vi "Calc_orders_FP.vi"() -> ()   [LabVIEW 2010]
panel:
  out "Phi Internal(deg)":dbl
  out "Pix rad (first ring)":dbl
  out "PhiExterna (deg)":dbl
  out "PhiExterna (rad)":dbl
  out "Phi Internal(rad)":dbl
  in  "order in":dbl=1100.0
  out "Angle (deg) cal-ed":dbl=9.9609375
  in  "rad first rimngs\n (pixels)":dbl=600.0
  out "gap (microns)":dbl=136.2709572898856
  in  "refractive index":dbl=3.4
  in  "Wavelength":dbl=1.2
  out "order":dbl=772.2020913093517
  out "cos(x)":dbl=0.9987050022121743
  out "sin(x)":dbl=0.050875520207473414
  in  "angle  (deg)":dbl=9.96094
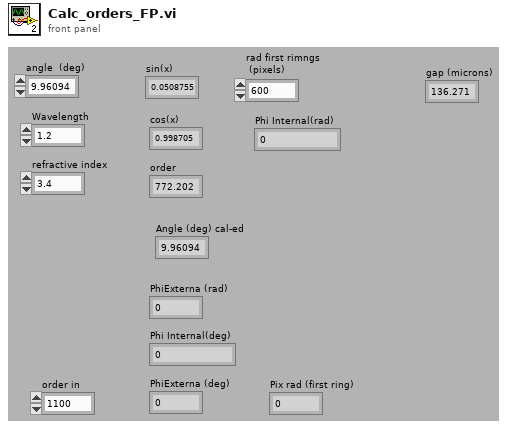
[diagram p1: front panel]
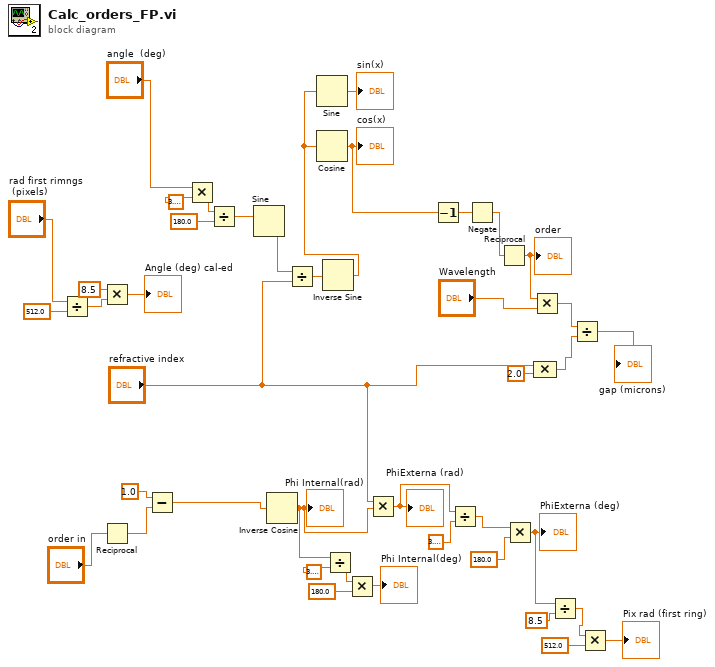
[diagram p0: block diagram]
diagram:
  n1 = Divide(x="rad first rimngs\n (pixels)", y=512.0) -> (x/y=w26:dbl)
  n2 = Multiply(x=8.5, y=w26) -> (x*y=→"Angle (deg) cal-ed":dbl)
  n3 = Reciprocal(x="order in") -> (1/x=w17:dbl)
  n4 = Subtract(x=1.0, y=w17) -> (x-y=w16:dbl)
  n5 = Multiply(x="angle  (deg)", y=3.141592653589793) -> (x*y=w36:dbl)
  n6 = Divide(x=w36, y=180.0) -> (x/y=w21:dbl)
  n7 = Sine(x=w21) -> (sin(x)=w22:dbl)
  n8 = Inverse Cosine(1:w16) -> (0:w2:dbl)
  "Phi Internal(rad)" <- w2
  n9 = Divide(x=w22, y="refractive index") -> (x/y=w23:dbl)
  n10 = Inverse Sine(1:w23) -> (0:w20:dbl)
  n11 = Sine(x=w20) -> (sin(x)=→"sin(x)":dbl)
  n12 = Cosine(x=w20) -> (cos(x)=w41:dbl)
  "cos(x)" <- w41
  n13 = Divide(x=w2, y=3.141592653589793) -> (x/y=w4:dbl)
  n14 = Multiply(x=w4, y=180.0) -> (x*y=→"Phi Internal(deg)":dbl)
  n15 = Multiply(x="refractive index", y=w2) -> (x*y=w9:dbl)
  "PhiExterna (rad)" <- w9
  n16 = Decrement(x=w41) -> (x-1=w40:dbl)
  n17 = Divide(x=w9, y=3.141592653589793) -> (x/y=w13:dbl)
  n18 = Negate(x=w40) -> (-x=w39:dbl)
  n19 = Reciprocal(x=w39) -> (1/x=w32:dbl)
  "order" <- w32
  n20 = Multiply(x=w13, y=180.0) -> (x*y=w8:dbl)
  "PhiExterna (deg)" <- w8
  n21 = Multiply(x=w32, y="Wavelength") -> (x*y=w30:dbl)
  n22 = Compound Arithmetic op=MULTIPLY("refractive index", 2.0 ("value")) -> (w29:dbl)
  n23 = Divide(x=w8, y=8.5 ("x")) -> (x/y=w7:dbl)
  n24 = Divide(x=w30, y=w29) -> (x/y=→"gap (microns)":dbl)
  n25 = Multiply(x=w7, y=512.0) -> (x*y=→"Pix rad (first ring)":dbl)
